vi "CRYCal TS Load.vi"(0 "Cal seq name":string) -> (7 "Cal sequence":T1 {"Steps"."Repeat State Array"."Start" format="%#_5g"; "Steps"."Y dB ref" format="%.1f"; "Steps"."Y data" items=["dB", "Lin"]; "Steps"."Start" format="%#_5g"}, 10 "status":bool)   [LabVIEW 2013]
uses:
  Typedef Control/CRYTS.ctl
  Typedef Control/CRYStep.ctl
  CRYMainGlobal.vi
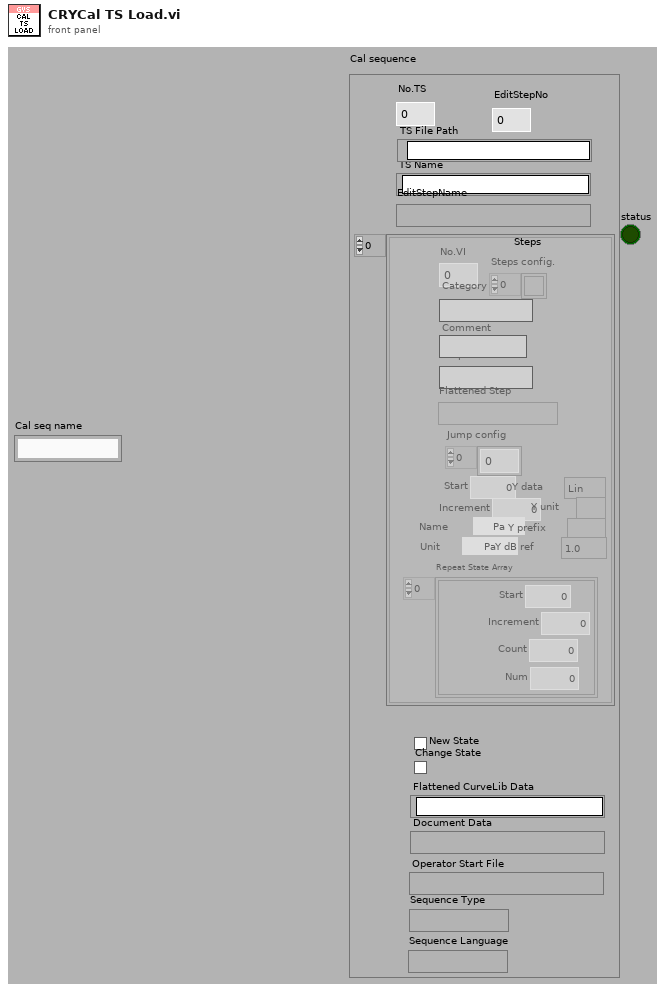
[diagram p1: front panel]
types:
  T1 = typedef "CRYTS.ctl" = cluster{"No.TS":u16, "TS File Path":path, "TS Name":string, "EditStepName":string, "Steps":T2[], "New State":bool, "Change State":bool, "Flattened CurveLib Data":string, "Document Data":string, "EditStepNo":u16, "Operator Start File":string, "Sequence Type":string, "Sequence Language":string}
  T2 = typedef "CRYStep.ctl" = cluster{"No.VI":i32, "Category":string, "StepName":string, "Seq setup flattened":string, "Comment":string, "Steps config.":bool[], "Jump config":i32[], "Start":dbl, "Increment":dbl, "Name":string, "Unit":string, "Y data":u16, "Y prefix":string, "Y dB ref":dbl, "Y unit":string, "Repeat State Array":cluster{"Start":dbl, "Increment":dbl, "Count":i32, "Num":i32}[]}
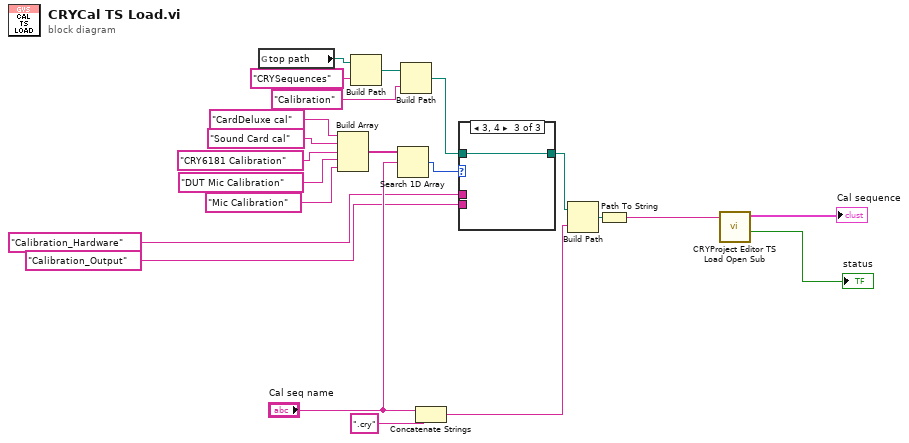
[diagram p0: block diagram]
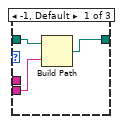
[diagram p2: hidden frame]
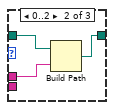
[diagram p3: hidden frame]
diagram:
  n1 = global read "CRYMainGlobal.vi" "top path"() -> (w17:path)
  n2 = Build Array("CardDeluxe cal", "Sound Card cal", "CRY6181 Calibration", "DUT Mic Calibration" ("y"), "Mic Calibration") -> (w14:string[])
  n3 = Build Path(base path=w17, name or relative path="CRYSequences") -> (appended path=w16:path)
  n4 = Search 1D Array(1D array=w14, element="Cal seq name") -> (index of element=w13:i32)  [unwired: 1 out]
  n5 = Build Path(base path=w16, name or relative path="Calibration") -> (appended path=w11:path)
  n6 = Concatenate Strings("Cal seq name", ".cry" ("regular expression")) -> (w19:string)
  n7 = case shown="3, 4" w13 {
    tunnel: w11 -> [w25 w28 w29]
    tunnel: [w23 w26 w29] -> w10
    tunnel: "Calibration_Hardware" ("name or relative path") -> [_ w27 _]
    tunnel: "Calibration_Output" ("name or relative path") -> [w24 _ _]
    frame -1, Default {
      n8 = Build Path(base path=w25, name or relative path=w24) -> (appended path=w23:path)
    }
    frame 0..2 {
      n9 = Build Path(base path=w28, name or relative path=w27) -> (appended path=w26:path)
    }
    frame 3, 4 {
    }
  }
  n10 = Build Path(base path=w10, name or relative path=w19) -> (appended path=w21:path)
  n11 = Path To String(path=w21) -> (string=w3:string)
  n12 = call "CRYProject Editor TS Load Open Sub.vi"("Seq File Name"=w3) -> ("TS Array"=→"Cal sequence":T1, "status"=→"status":bool)  [unwired: 8 in]
